vi "COMI Write EEPR.vi"(9 "data":i32, 10 "addr":i32, 11 "hDevice":u32) -> (3 "hDevice out":u32)   [LabVIEW 2017, in "Comidll.lvlib"]
doc: "void (COMI_WriteEEPR) (HANDLE hDevice, int addr, int data);"
uses:
  <userlib>/Comidll/Comidll.lvlib
  <userlib>/Comidll/Comidll.dll
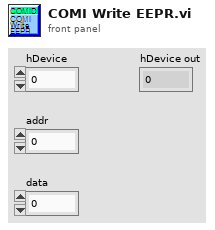
[diagram p1: front panel]
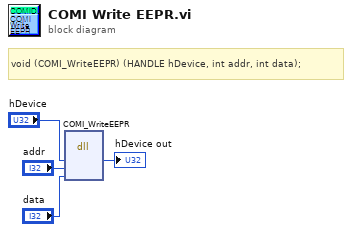
[diagram p0: block diagram]
diagram:
  # "void\t(COMI_WriteEEPR) (HANDLE hDevice, int addr, int data);"
  n1 = dll-call lib="C:/Program Files/National Instruments/LabVIEW 2017/user.lib/Comidll/Comidll.*" fn="COMI_WriteEEPR"("hDevice"="hDevice", "addr"="addr", "data"="data") -> ("hDevice"=→"hDevice out":u32)  [unwired: 6 in, 2 out]
